vi "rolamento_interno.vi"   [LabVIEW 2020]
uses:
  <vilib>/Rock Robotics/WPI/ThirdParty/Phoenix-LabVIEW/Motor Controller/Controls/CTRE_Phoenix_MotorControl_ControlMode.ctl
  GlobalVariables.vi
types:
  T1 = cluster{"POVs[0]":i16, "POVs[1]":i16, "POVs[2]":i16, "POVs[3]":i16, "POVs[4]":i16, "POVs[5]":i16, "POVs[6]":i16, "POVs[7]":i16}
  T2 = typedef "CTRE_Phoenix_MotorControl_ControlMode.ctl" = u16
  T3 = typedef "WPI_MotorControlDeviceRef.ctl" = cluster{"DeviceStatus":errorcluster, "Type":T4, "PWM":cluster{"PWM Channel":T5, "DeadBand":T6}, "CAN":cluster{"Device Number":u8, "SetOutput VI Ref":variant, "GetOutput VI Ref":variant, "Enable VI Ref":variant, "Disable VI Ref":variant, "Data":variant}, "Invert":bool, "DIO PWM":cluster{"PWM \"Enable\" Channel":T5, "DIOChannel":T7, "PWM Rate":dbl}}
  T4 = typedef "WPI_MotorControlType.ctl" = enum16{"PWM", "CAN", "DIO PWM"}
  T5 = typedef "FPGA_DIOPWMChannel.ctl" = enum8{"PWM 0", "PWM 1", "PWM 2", "PWM 3", "PWM 4", "PWM 5", "PWM 6", "PWM 7", "PWM 8", "PWM 9", "PWM MXP 0", "PWM MXP 1", "PWM MXP 2", "PWM MXP 3", "PWM MXP 4", "PWM MXP 5", "PWM MXP 6", "PWM MXP 7", "PWM MXP 8", "PWM MXP 9", "Invalid"}
  T6 = typedef "WPI_PWMDeadband.ctl" = cluster{"Name":string, "maxPositivePwm":i32, "minPositivePwm":i32, "centerPwm":i32, "maxNegativePwm":i32, "minNegativePwm":i32, "angularRange":u16}
  T7 = typedef "FPGA_DIOChannel.ctl" = enum8{"DIO 0", "DIO 1", "DIO 2", "DIO 3", "DIO 4", "DIO 5", "DIO 6", "DIO 7", "DIO 8", "DIO 9", "DIO MXP 0", "DIO MXP 1", "DIO MXP 2", "DIO MXP 3", "DIO MXP 4", "DIO MXP 5", "DIO MXP 6", "DIO MXP 7", "DIO MXP 8", "DIO MXP 9", "DIO MXP 10", "DIO MXP 11", "DIO MXP 12", "DIO MXP 13", "DIO MXP 14", "DIO MXP 15", "SPI Port CS1", "SPI Port CS2", "SPI Port CS3", "SPI Port MISO", "SPI Port MOSI", "Invalid"}
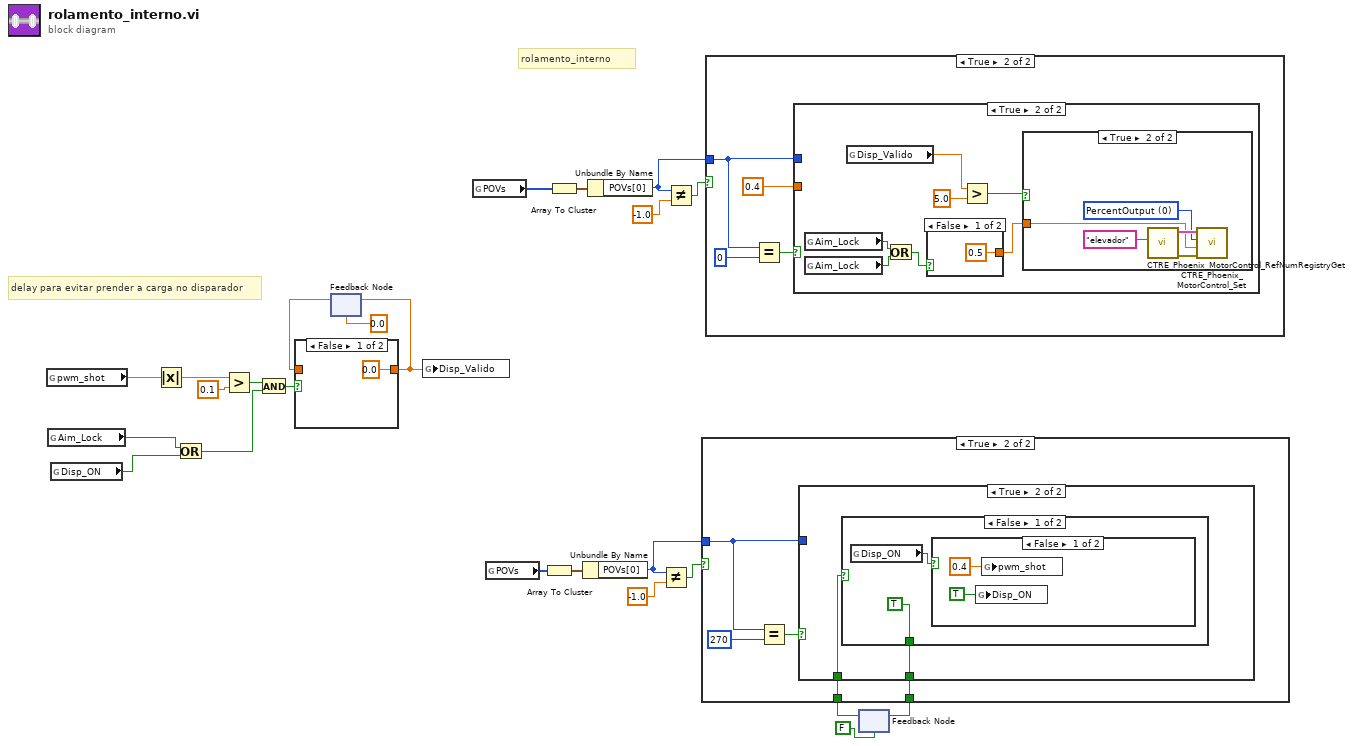
[diagram p0: block diagram]
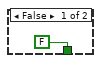
[diagram p2: hidden frame]
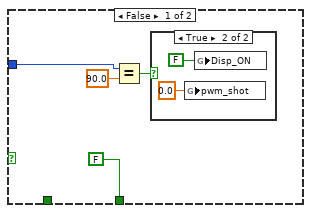
[diagram p3: hidden frame]
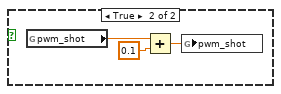
[diagram p5: hidden frame]
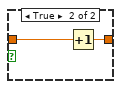
[diagram p7: hidden frame]
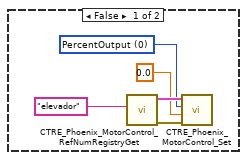
[diagram p8: hidden frame]
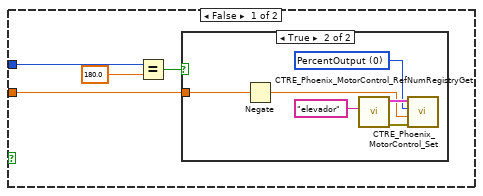
[diagram p9: hidden frame]
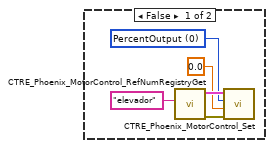
[diagram p10: hidden frame]
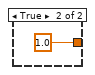
[diagram p11: hidden frame]
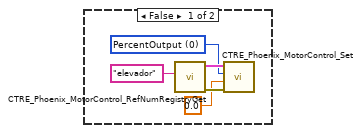
[diagram p12: hidden frame]
diagram:
  # "delay para evitar prender a carga no disparador"
  # "rolamento_interno"
  n1 = global read "GlobalVariables.vi" "pwm_shot"() -> (w13:dbl)
  n2 = global read "GlobalVariables.vi" "Aim_Lock"() -> (w10:bool)
  n3 = global read "GlobalVariables.vi" "Disp_ON"() -> (w9:bool)
  n4 = Absolute Value(x=w13) -> (abs(x)=w19:dbl)
  n5 = Or(x=w10, y=w9) -> (x .or. y?=w11:bool)
  n6 = Greater?(x=w19, y=0.1) -> (0:w18:bool)
  n7 = And(x=w18, y=w11) -> (x .and. y?=w17:bool)
  n8 = feedback #1(0.0) -> (w15:dbl)
  n9 = case shown="False" w17 {
    tunnel: [0.0 w27] -> w12
    tunnel: w15 -> [_ w26]
    frame False {
    }
    frame True {
      n10 = Increment(x=w26) -> (x+1=w27:dbl)
    }
  }
  n11 = feedback-in #1(w12) -> ()
  n12 = global write "GlobalVariables.vi" "Disp_Valido"(w12) -> ()
  n13 = global read "GlobalVariables.vi" "POVs"() -> (w14:i16[])
  n14 = global read "GlobalVariables.vi" "POVs"() -> (w4:i16[])
  n15 = Array To Cluster(array=w4) -> (cluster=w6:T1)
  n16 = Array To Cluster(array=w14) -> (cluster=w22:T1)
  n17 = Unbundle By Name(w6) -> ("POVs[0]"=w5:i16)
  n18 = Unbundle By Name(w22) -> ("POVs[0]"=w21:i16)
  n19 = Not Equal?(x=w5, y=-1.0) -> (x != y?=w7:bool)
  n20 = Not Equal?(x=w21, y=-1.0) -> (x != y?=w23:bool)
  n21 = case shown="True" w23 {
    tunnel: w21 -> [_ w34]
    frame False {
      w29 = T2 0 items=["PercentOutput"=0, "Position"=1, "Velocity"=2, "Current"=3, "Follower"=5, "MotionProfile"=6, "MotionMagic"=7, "MotionProfileArc"=10, "Disabled"=15] ("Control Mode")
      n22 = call <vilib>:"CTRE_Phoenix_MotorControl_RefNumRegistryGet.vi"("refnum name"="elevador") -> ("error out"=w31:errorcluster, "PhoenixMotorControlDevRef"=w32:T3)  [unwired: 9 in]
      n23 = call <vilib>:"CTRE_Phoenix_MotorControl_Set.vi"("error in (no error)"=w31, "Output"=0.0, "Control Mode"=w29, "PhoenixMotorControlDevRef"=w32) -> ()  [unwired: 6 in, 2 out]
    }
    frame True {
      n24 = Equal?(x=w34, y=i16 0) -> (x = y?=w35:bool)
      n25 = case shown="True" w35 {
        tunnel: w34 -> [w38 _]
        tunnel: 0.4 ("Output") -> [w37 _]
        frame False {
          n26 = Equal?(x=w38, y=180.0) -> (x = y?=w40:bool)
          n27 = case shown="True" w40 {
            tunnel: w37 -> [_ w46]
            frame False {
              w43 = T2 0 items=["PercentOutput"=0, "Position"=1, "Velocity"=2, "Current"=3, "Follower"=5, "MotionProfile"=6, "MotionMagic"=7, "MotionProfileArc"=10, "Disabled"=15] ("Control Mode")
              n28 = call <vilib>:"CTRE_Phoenix_MotorControl_RefNumRegistryGet.vi"("refnum name"="elevador") -> ("error out"=w44:errorcluster, "PhoenixMotorControlDevRef"=w45:T3)  [unwired: 9 in]
              n29 = call <vilib>:"CTRE_Phoenix_MotorControl_Set.vi"("error in (no error)"=w44, "Output"=0.0, "Control Mode"=w43, "PhoenixMotorControlDevRef"=w45) -> ()  [unwired: 6 in, 2 out]
            }
            frame True {
              w49 = T2 0 items=["PercentOutput"=0, "Position"=1, "Velocity"=2, "Current"=3, "Follower"=5, "MotionProfile"=6, "MotionMagic"=7, "MotionProfileArc"=10, "Disabled"=15] ("Control Mode")
              n30 = Negate(x=w46) -> (-x=w47:dbl)
              n31 = call <vilib>:"CTRE_Phoenix_MotorControl_RefNumRegistryGet.vi"("refnum name"="elevador") -> ("error out"=w50:errorcluster, "PhoenixMotorControlDevRef"=w51:T3)  [unwired: 9 in]
              n32 = call <vilib>:"CTRE_Phoenix_MotorControl_Set.vi"("error in (no error)"=w50, "Output"=w47, "Control Mode"=w49, "PhoenixMotorControlDevRef"=w51) -> ()  [unwired: 6 in, 2 out]
            }
          }
        }
        frame True {
          n33 = global read "GlobalVariables.vi" "Aim_Lock"() -> (w54:bool)
          n34 = global read "GlobalVariables.vi" "Aim_Lock"() -> (w53:bool)
          n35 = global read "GlobalVariables.vi" "Disp_Valido"() -> (w55:dbl)
          n36 = Or(x=w54, y=w53) -> (x .or. y?=w52:bool)
          n37 = case shown="False" w52 {
            tunnel: [0.5 ("Output") 1.0 ("Output")] -> w56
            frame False {
            }
            frame True {
            }
          }
          n38 = Greater?(x=w55, y=5.0) -> (0:w58:bool)
          n39 = case shown="True" w58 {
            tunnel: w56 -> [_ w66]
            frame False {
              w63 = T2 0 items=["PercentOutput"=0, "Position"=1, "Velocity"=2, "Current"=3, "Follower"=5, "MotionProfile"=6, "MotionMagic"=7, "MotionProfileArc"=10, "Disabled"=15] ("Control Mode")
              n40 = call <vilib>:"CTRE_Phoenix_MotorControl_RefNumRegistryGet.vi"("refnum name"="elevador") -> ("error out"=w64:errorcluster, "PhoenixMotorControlDevRef"=w65:T3)  [unwired: 9 in]
              n41 = call <vilib>:"CTRE_Phoenix_MotorControl_Set.vi"("error in (no error)"=w64, "Output"=0.0, "Control Mode"=w63, "PhoenixMotorControlDevRef"=w65) -> ()  [unwired: 6 in, 2 out]
            }
            frame True {
              w68 = T2 0 items=["PercentOutput"=0, "Position"=1, "Velocity"=2, "Current"=3, "Follower"=5, "MotionProfile"=6, "MotionMagic"=7, "MotionProfileArc"=10, "Disabled"=15] ("Control Mode")
              n42 = call <vilib>:"CTRE_Phoenix_MotorControl_RefNumRegistryGet.vi"("refnum name"="elevador") -> ("error out"=w69:errorcluster, "PhoenixMotorControlDevRef"=w70:T3)  [unwired: 9 in]
              n43 = call <vilib>:"CTRE_Phoenix_MotorControl_Set.vi"("error in (no error)"=w69, "Output"=w66, "Control Mode"=w68, "PhoenixMotorControlDevRef"=w70) -> ()  [unwired: 6 in, 2 out]
            }
          }
        }
      }
    }
  }
  n44 = feedback #2(FALSE) -> (w2:bool)
  n45 = case shown="True" w7 {
    tunnel: w5 -> [_ w74]
    tunnel: w2 -> [_ w73]
    tunnel: [FALSE w72] -> w1
    frame False {
    }
    frame True {
      n46 = Equal?(x=w74, y=i16 270) -> (x = y?=w75:bool)
      n47 = case shown="True" w75 {
        tunnel: w74 -> [w78 _]
        tunnel: w73 -> [_ w84]
        tunnel: [FALSE w83] -> w72
        frame False {
          n48 = Equal?(x=w78, y=90.0) -> (x = y?=w80:bool)
          n49 = case shown="True" w80 {
            frame False {
            }
            frame True {
              n50 = global write "GlobalVariables.vi" "pwm_shot"(0.0 ("pwm_shot")) -> ()
              n51 = global write "GlobalVariables.vi" "Disp_ON"(FALSE ("Disp_ON")) -> ()
            }
          }
        }
        frame True {
          n52 = case shown="False" w84 {
            selector: w84 -> [_ w92]
            tunnel: [TRUE w92] -> w83
            frame False {
              n53 = global read "GlobalVariables.vi" "Disp_ON"() -> (w86:bool)
              n54 = case shown="False" w86 {
                frame False {
                  n55 = global write "GlobalVariables.vi" "Disp_ON"(TRUE) -> ()
                  n56 = global write "GlobalVariables.vi" "pwm_shot"(0.4) -> ()
                }
                frame True {
                  n57 = global read "GlobalVariables.vi" "pwm_shot"() -> (w91:dbl)
                  n58 = Add(x=w91, y=0.1) -> (x+y=w90:dbl)
                  n59 = global write "GlobalVariables.vi" "pwm_shot"(w90) -> ()
                }
              }
            }
            frame True {
            }
          }
        }
      }
    }
  }
  n60 = feedback-in #2(w1) -> ()
